vi "Multiply - CM,C.vi"(1 "Complex Scalar c":cdb, 2 "Complex Matrix A":T1) -> (0 "A * c":T1)   [LabVIEW 2014, in "NI_Matrix.lvlib"]
doc: "Returns the product of the inputs."
uses:
  NI_Matrix.lvlib
  ComplexMatrix.ctl
  Array To Matrix - CA2.vi
  Matrix To Array - CM.vi
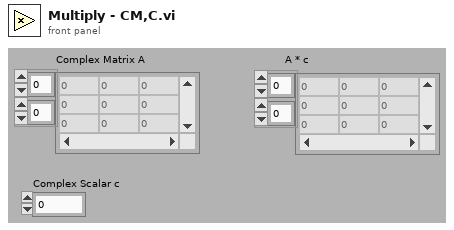
[diagram p1: front panel]
types:
  T1 = typedef "NI_Matrix.lvlib/ComplexMatrix.ctl" = cdb[][]
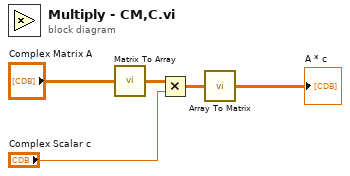
[diagram p0: block diagram]
diagram:
  n1 = call-poly "Matrix To Array.vi"("Complex Matrix"="Complex Matrix A") -> ("Complex 2D Array"=w4:cdb[][])
  n2 = Multiply(x=w4, y="Complex Scalar c") -> (x*y=w2:cdb[][])
  n3 = call-poly "Array To Matrix.vi"("Complex 2D Array"=w2) -> ("Complex Matrix"=→"A * c":T1)
